vi "Save File Parse Software Version.vi"(11 "Message":string) -> (3 "UI Version":T1)   [LabVIEW 2016, in "Save File.lvlib"]
uses:
  Save File.lvlib
  Type Definitions/Save File Software Version.ctl
  LabVIEW GEA2 Toolkit v1.0.0.0/library/GEA2_Toolkit.lvlib
panel:
  # "01 01 01 29 00 00"
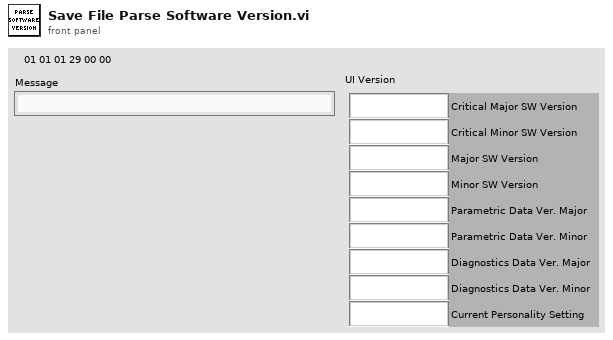
[diagram p1: front panel]
types:
  T1 = typedef "Save File.lvlib/Save File Software Version.ctl" = cluster{"Critical Major SW Version":string, "Critical Minor SW Version":string, "Major SW Version":string, "Minor SW Version":string, "Parametric Data Ver. Major":string, "Parametric Data Ver. Minor":string, "Diagnostics Data Ver. Major":string, "Diagnostics Data Ver. Minor":string, "Current Personality Setting":string}
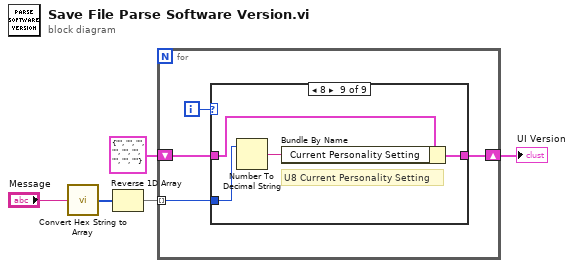
[diagram p0: block diagram]
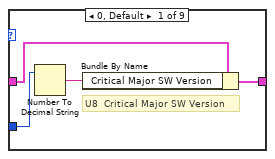
[diagram p2: hidden frame]
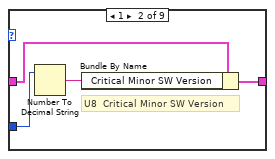
[diagram p3: hidden frame]
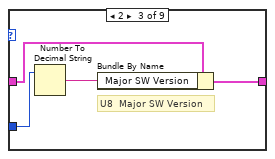
[diagram p4: hidden frame]
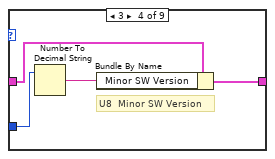
[diagram p5: hidden frame]
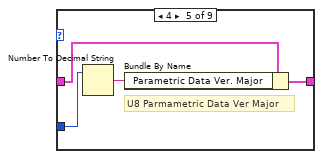
[diagram p6: hidden frame]
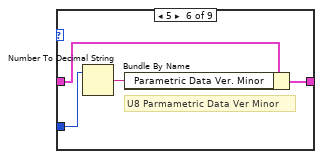
[diagram p7: hidden frame]
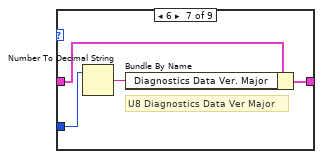
[diagram p8: hidden frame]
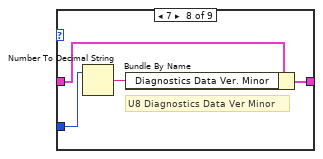
[diagram p9: hidden frame]
diagram:
  n1 = call "Convert Hex String to Array.vi"("Hex String In"="Message") -> ("Hex Array Out"=w2:u8[])  [unwired: 14 in]
  n2 = Reverse 1D Array(array=w2) -> (reversed array=w1:u8[])
  n3 = for {
    tunnel: w1 -> [w8] mode=indexing
    shift-right: [w6] -> w4
    shift-left: T1 {"Critical Major SW Version"="", "Critical Minor SW Version"="", "Major SW Version"="", "Minor SW Version"="", "Parametric Data Ver. Major"="", "Parametric Data Ver. Minor"="", "Diagnostics Data Ver. Major"="", "Diagnostics Data Ver. Minor"="", "Current Personality Setting"=""} ("UI Version 2") -> [w7]
    i -> [w9]
    n4 = case shown="8" w9 {
      tunnel: w8 -> [w13 w16 w21 w24 w28 w32 w36 w40 w44]
      tunnel: w7 -> [w12 w15 w19 w23 w27 w31 w35 w39 w43]
      tunnel: [w10 w14 w18 w22 w26 w30 w34 w38 w42] -> w6
      frame 0, Default {
        # "U8  Critical Major SW Version"
        n5 = Number To Decimal String(number=w13) -> (decimal integer string=w11:string)  [unwired: 1 in]
        n6 = Bundle By Name(cluster=w12, "Critical Major SW Version"=w11) -> (w10:T1)
      }
      frame 1 {
        # "U8  Critical Minor SW Version"
        n7 = Number To Decimal String(number=w16) -> (decimal integer string=w17:string)  [unwired: 1 in]
        n8 = Bundle By Name(cluster=w15, "Critical Minor SW Version"=w17) -> (w14:T1)
      }
      frame 2 {
        # "U8  Major SW Version"
        n9 = Number To Decimal String(number=w21) -> (decimal integer string=w20:string)  [unwired: 1 in]
        n10 = Bundle By Name(cluster=w19, "Major SW Version"=w20) -> (w18:T1)
      }
      frame 3 {
        # "U8  Minor SW Version"
        n11 = Number To Decimal String(number=w24) -> (decimal integer string=w25:string)  [unwired: 1 in]
        n12 = Bundle By Name(cluster=w23, "Minor SW Version"=w25) -> (w22:T1)
      }
      frame 4 {
        # "U8 Parmametric Data Ver Major"
        n13 = Number To Decimal String(number=w28) -> (decimal integer string=w29:string)  [unwired: 1 in]
        n14 = Bundle By Name(cluster=w27, "Parametric Data Ver. Major"=w29) -> (w26:T1)
      }
      frame 5 {
        # "U8 Parmametric Data Ver Minor"
        n15 = Number To Decimal String(number=w32) -> (decimal integer string=w33:string)  [unwired: 1 in]
        n16 = Bundle By Name(cluster=w31, "Parametric Data Ver. Minor"=w33) -> (w30:T1)
      }
      frame 6 {
        # "U8 Diagnostics Data Ver Major"
        n17 = Number To Decimal String(number=w36) -> (decimal integer string=w37:string)  [unwired: 1 in]
        n18 = Bundle By Name(cluster=w35, "Diagnostics Data Ver. Major"=w37) -> (w34:T1)
      }
      frame 7 {
        # "U8 Diagnostics Data Ver Minor"
        n19 = Number To Decimal String(number=w40) -> (decimal integer string=w41:string)  [unwired: 1 in]
        n20 = Bundle By Name(cluster=w39, "Diagnostics Data Ver. Minor"=w41) -> (w38:T1)
      }
      frame 8 {
        # "U8 Current Personality Setting"
        n21 = Number To Decimal String(number=w44) -> (decimal integer string=w45:string)  [unwired: 1 in]
        n22 = Bundle By Name(cluster=w43, "Current Personality Setting"=w45) -> (w42:T1)
      }
    }
  }
  "UI Version" <- w4
